vi "OFF_Polarity_Channel_ALLSET_minGain.vi"(5 "CH_ON:0/OFF:1":u16, 7 "Mode":u16(ring)=1 items=["Tx"=1, "Rx"=2], 8 "error in":errorcluster, 10 "Channel":i32=64, 11 "TCPIPin":T1={"address"="192.168.100.111", "remote port or service name"=5025, "timeout ms (60000)"=10000}) -> (0 "error out":errorcluster, 1 "OK?":bool, 3 "TCPIPout":T1={"address"="192.168.100.111", "remote port or service name"=5025, "timeout ms (60000)"=10000})   [LabVIEW 2023]
panel:
  out "Array":string[][](array[string])
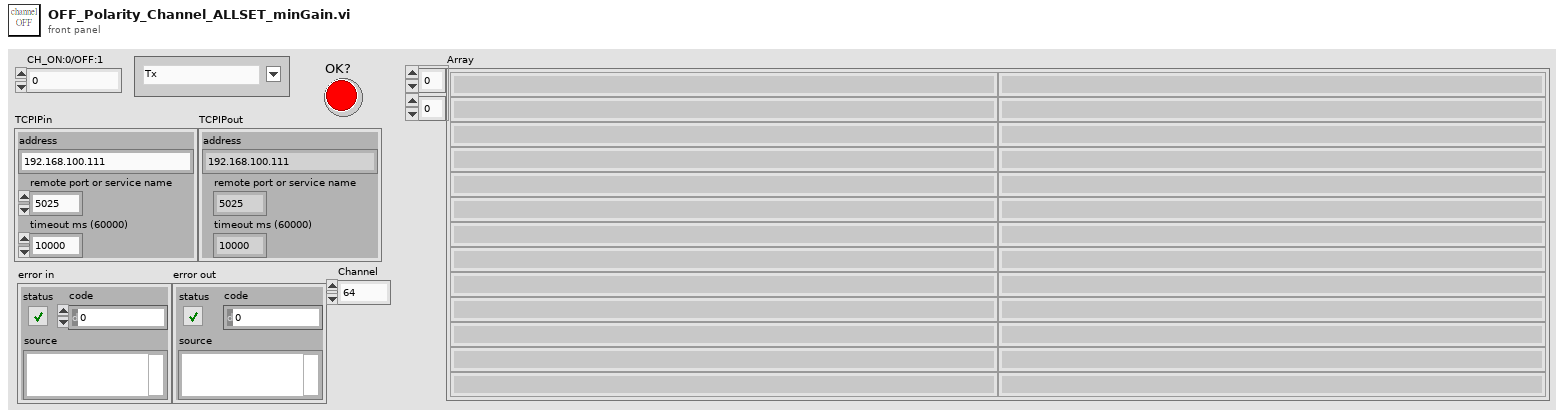
[diagram p1: front panel]
types:
  T1 = cluster{"address":string, "remote port or service name":u16, "timeout ms (60000)":i32}
  T2 = cluster{"Mode":u16, "Polarity":u16, "CH_ON/OFF":u16, "Channel":i32, "Gain":i32, "Phase":i32}
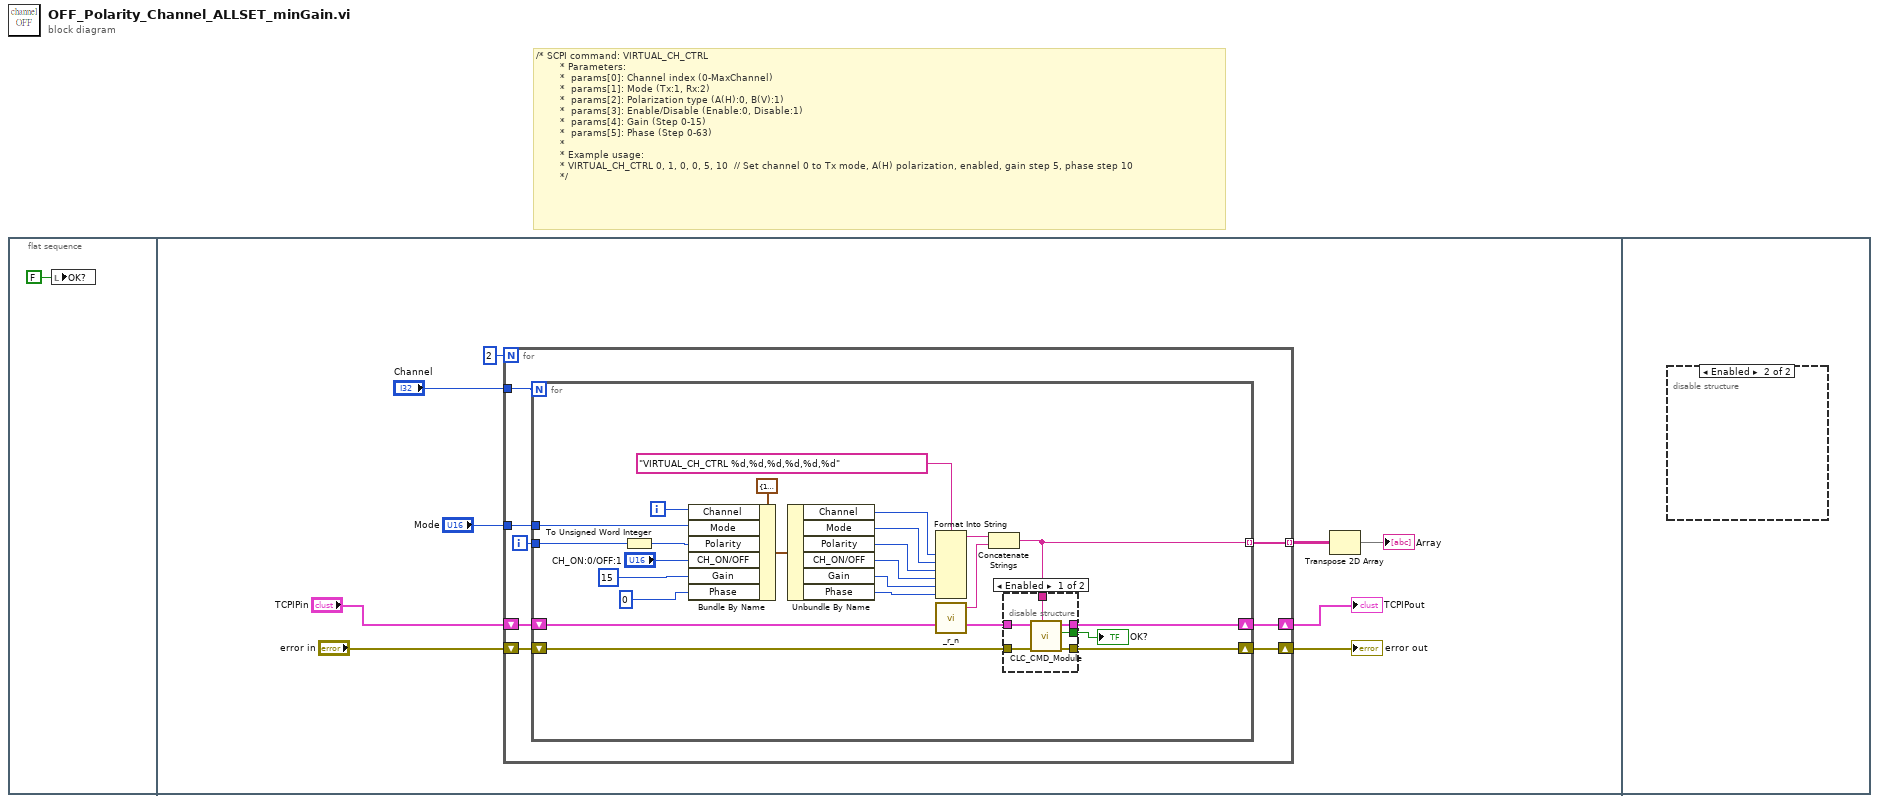
[diagram p0: block diagram]
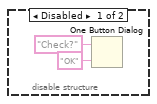
[diagram p3: hidden frame]
diagram:
  # "/* SCPI command: VIRTUAL_CH_CTRL\n        * Parameters:\n        *  params[0]: Channel index (0-MaxChannel)\n        *  params[1]: Mode (Tx:1, Rx:2)\n        *  params[2]: Polarization type (A(H):0, B(V):1)\n        *  params[3]: Enable/Disable (Enable:0, Disable:1)\n        *  params[4]: Gain (Step 0-15)\n        *  params[5]: Phase (Step 0-63)\n        * \n        * Example usage:\n        * VIRTUAL_CH_CTRL 0, 1, 0, 0, 5, 10  // Set channel 0 to Tx mode, A(H) polarization, enabled, gain step 5, phase step 10\n        */"
  n1 = flat-sequence {
    frame #0 {
      n2 = local write "OK?"(FALSE ("OK?")) -> ()
    }
    frame #1 {
      n3 = for {
        N: 2 -> [_]
        shift-right: [w17] -> w9
        shift-left: "TCPIPin" -> [w18]
        shift-right: [w15] -> w7
        shift-left: "error in" -> [w16]
        tunnel: "Mode" -> [w14]
        tunnel: [w12] -> w4 mode=indexing
        tunnel: "Channel" -> [w11]
        i -> [w13]
        n4 = for {
          N: w11 -> [_]
          shift-right: [w41] -> w17
          shift-left: w18 -> [w42]
          shift-right: [w39] -> w15
          shift-left: w16 -> [w40]
          tunnel: w14 -> [w27]
          tunnel: w13 -> [w24]
          tunnel: [w21] -> w12 mode=indexing
          i -> [w25]
          n5 = To Unsigned Word Integer(number=w24) -> (unsigned 16bit integer=w23:u16)
          n6 = Bundle By Name(cluster=T2 {"Mode"=1, "Polarity"=1, "CH_ON/OFF"=1, "Channel"=0, "Gain"=0, "Phase"=0} ("Channel params"), "Channel"=w25, "Mode"=w27, "Polarity"=w23, "CH_ON/OFF"="CH_ON:0/OFF:1", "Gain"=15, "Phase"=0) -> (w28:T2)
          n7 = Unbundle By Name(w28) -> ("Channel"=w33:i32, "Mode"=w34:u16, "Polarity"=w35:u16, "CH_ON/OFF"=w36:u16, "Gain"=w37:i32, "Phase"=w38:i32)
          n8 = Format Into String(format string="VIRTUAL_CH_CTRL %d,%d,%d,%d,%d,%d" ("data in"), w33, w34, w35, w36, w37, w38) -> (resulting string=w31:string)  [unwired: 2 in, 1 out]
          n9 = call "_r_n.vi"() -> ("command"=w32:string)  [unwired: 5 in]
          n10 = Concatenate Strings(w31, w32) -> (w21:string)
          n11 = disable-structure shown="Enabled" {
            disable-tunnel: w42 -> [w48 w50]
            disable-tunnel: [w47 w50] -> w41
            disable-tunnel: w40 -> [w46 w49]
            disable-tunnel: [w45 w49] -> w39
            disable-tunnel: w21 -> [w44 _]
            disable-tunnel: [w43 _] -> w26
            frame Enabled {
              n12 = call "CLC_CMD_Module.vi"("CMD in"=w44, "error in"=w46, "TCPIPin"=w48) -> ("error out"=w45:errorcluster, "OK?"=w43:bool, "TCPIPout"=w47:T1)  [unwired: 5 in, 1 out]
            }
            frame Disabled {
            }
          }
          "OK?" <- w26
        }
      }
      "TCPIPout" <- w9
      "error out" <- w7
      n13 = Transpose 2D Array(2D array=w4) -> (transposed array=→"Array":string[][])
    }
    frame #2 {
      n14 = disable-structure shown="Enabled" {
        frame Disabled {
          n15 = One Button Dialog(message="Check?", button name ("OK")="OK") -> ()  [unwired: 1 out]
        }
        frame Enabled {
        }
      }
    }
  }
